vi "Find Distance.vi"(8 "error in (no error)":errorcluster, 9 "Direction":T1, 10 "Position":T2, 11 "Maze in":refnum<class "Maze.lvclass">) -> (0 "error out":errorcluster, 2 "Distance":i32)   [LabVIEW 2020, in "Maze.lvlib" / "Maze.lvclass"]
uses:
  Maze.lvclass
  Position.ctl
  Direction.ctl
  Maze.lvclass/Maze.ctl
  Maze.lvlib
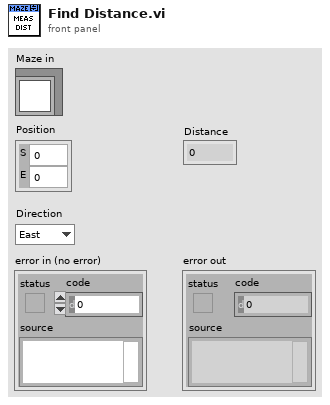
[diagram p1: front panel]
types:
  T1 = typedef "Maze.lvlib/Direction.ctl" = enum8{"East", "North", "West", "South"}
  T2 = typedef "Maze.lvlib/Position.ctl" = cluster{"S":i32, "E":i32}
  T3 = typedef "Maze.lvlib/Adjacency.ctl" = cluster{"E":bool, "N":bool, "W":bool, "S":bool, "Goal":bool, "Start":bool}
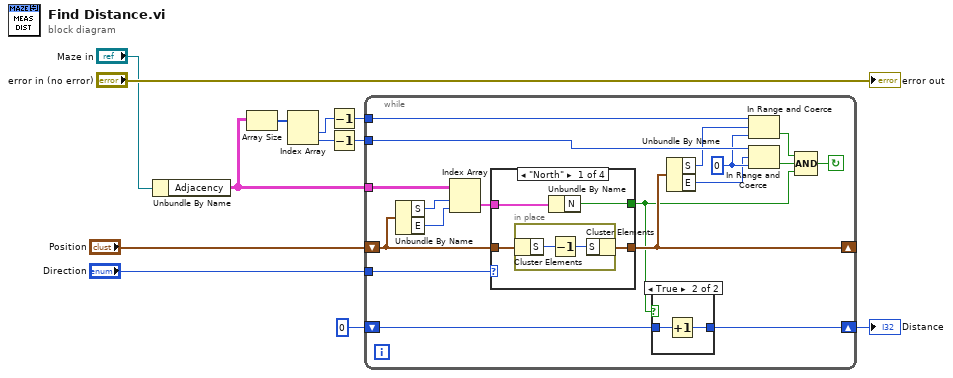
[diagram p0: block diagram]
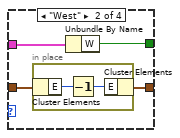
[diagram p3: hidden frame]
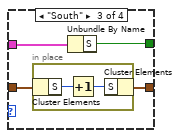
[diagram p4: hidden frame]
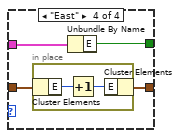
[diagram p5: hidden frame]
diagram:
  n1 = Unbundle By Name("Maze in") -> ("Adjacency"=w7:T3[][])
  n2 = Array Size(array=w7) -> (size(s)=w6:i32[])
  n3 = Index Array(array=w6) -> (element #1=w5:i32, element #2=w3:i32)  [unwired: 2 in]
  n4 = Decrement(x=w5) -> (x-1=w4:i32)
  n5 = Decrement(x=w3) -> (x-1=w2:i32)
  n6 = while {
    tunnel: w7 -> [w30]
    shift-right: [w19] -> _
    shift-left: "Position" -> [w26]
    tunnel: "Direction" -> [w25]
    shift-right: [w23] -> w1
    shift-left: 0 -> [w24]
    tunnel: w4 -> [w22]
    tunnel: w2 -> [w21]
    stop <- w13 continue-if-true
    w20 = 0 ("lower limit")
    n7 = Unbundle By Name(w26) -> ("S"=w29:i32, "E"=w28:i32)
    n8 = Index Array(array=w30, index (row)=w29, index (col)=w28) -> (element=w27:T3)
    n9 = case shown="\"North\"" w25 {
      tunnel: w27 -> [w35 w41 w47 w53]
      tunnel: w26 -> [w37 w43 w49 w55]
      tunnel: [w36 w42 w48 w54] -> w19
      tunnel: [w34 w40 w46 w52] -> w14
      frame "North" {
        n10 = in-place {
          n11 = in-place-cluster #1(w37) -> ("S"=w39:i32)
          n12 = Decrement(x=w39) -> (x-1=w38:i32)
          n13 = in-place-cluster #1("S"=w38) -> (w36:T2)
        }
        n14 = Unbundle By Name(w35) -> ("N"=w34:bool)
      }
      frame "West" {
        n15 = in-place {
          n16 = in-place-cluster #2(w43) -> ("E"=w45:i32)
          n17 = Decrement(x=w45) -> (x-1=w44:i32)
          n18 = in-place-cluster #2("E"=w44) -> (w42:T2)
        }
        n19 = Unbundle By Name(w41) -> ("W"=w40:bool)
      }
      frame "South" {
        n20 = in-place {
          n21 = in-place-cluster #3(w49) -> ("S"=w51:i32)
          n22 = Increment(x=w51) -> (x+1=w50:i32)
          n23 = in-place-cluster #3("S"=w50) -> (w48:T2)
        }
        n24 = Unbundle By Name(w47) -> ("S"=w46:bool)
      }
      frame "East" {
        n25 = in-place {
          n26 = in-place-cluster #4(w55) -> ("E"=w57:i32)
          n27 = Increment(x=w57) -> (x+1=w56:i32)
          n28 = in-place-cluster #4("E"=w56) -> (w54:T2)
        }
        n29 = Unbundle By Name(w53) -> ("E"=w52:bool)
      }
    }
    n30 = case shown="True" w14 {
      tunnel: w24 -> [w31 w33]
      tunnel: [w31 w32] -> w23
      frame False {
      }
      frame True {
        n31 = Increment(x=w33) -> (x+1=w32:i32)
      }
    }
    n32 = Unbundle By Name(w19) -> ("S"=w18:i32, "E"=w17:i32)
    n33 = In Range and Coerce(upper limit=w22, x=w18, lower limit=w20) -> (In Range?=w15:bool)  [unwired: 1 out]
    n34 = In Range and Coerce(upper limit=w21, x=w17, lower limit=w20) -> (In Range?=w16:bool)  [unwired: 1 out]
    n35 = Compound Arithmetic op=AND(w15, w16, w14) -> (w13:bool)
  }
  "Distance" <- w1
  "error out" <- "error in (no error)"
